vi "Com ID Check.vi"(8 "error in (no error)":errorcluster, 11 "VISA Refnum in":refnum<visa-resource-name>) -> (0 "error out":errorcluster, 3 "VISA Refnum out":refnum<visa-resource-name>)   [LabVIEW 2016, in "SR7270 Drivers.lvclass"]
uses:
  SR7270 Drivers.lvclass
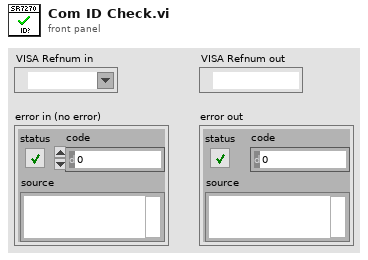
[diagram p1: front panel]
types:
  T1 = cluster{"status":bool, "code":i32, "SR 7124 Initialize":string}
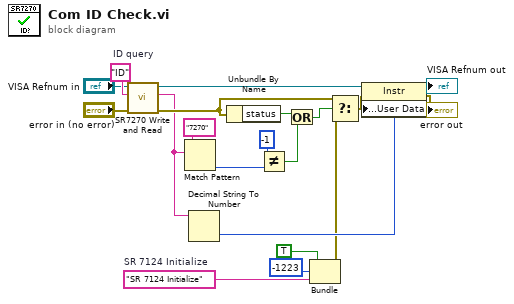
[diagram p0: block diagram]
diagram:
  w18 = "SR 7124 Initialize"  # SR 7124 Initialize
  w14 = "ID"  # ID query
  n1 = call "SR7270 Write and Read.vi"("error in (no error)"="error in (no error)", "Command Name"=w14, "VISA resource name"="VISA Refnum in") -> ("error out"=w17:errorcluster, "Read"=w15:string, "VISA resource name out"=w12:refnum<visa-resource-name>)  [unwired: 5 in, 1 out]
  n2 = Match Pattern(string=w15, regular expression="7270") -> (offset past match=w4:i32)  [unwired: 1 in, 3 out]
  n3 = Decimal String To Number(string=w15) -> (number=w19:i32)  [unwired: 2 in, 1 out]
  n4 = Unbundle By Name(w17) -> ("status"=w6:bool)
  n5 = Not Equal?(x=-1, y=w4) -> (x != y?=w7:bool)
  n6 = Or(x=w6, y=w7) -> (x .or. y?=w16:bool)
  n7 = Bundle(TRUE, -1223, "SR 7124 Initialize"=w18) -> (w3:cluster{bool, i32, "SR 7124 Initialize":string})  [unwired: 1 in]
  n8 = Select(t=w17, s=w16, f=w3) -> (s? t:f=w9:T1)
  n9 = property class="Instr"(reference=w12, error in=w9, "General Settings:User Data"=w19) -> (reference out=→"VISA Refnum out":refnum<visa-resource-name>, error out=→"error out":errorcluster)
